vi "BoolDebExample.vi"() -> ()   [LabVIEW 2012]
panel:
  in  "stop":bool
  in  "Default":bool
  out "Boolean 2":bool
  in  "Boolean":bool
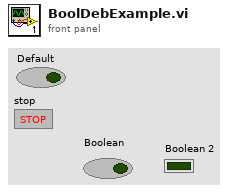
[diagram p1: front panel]
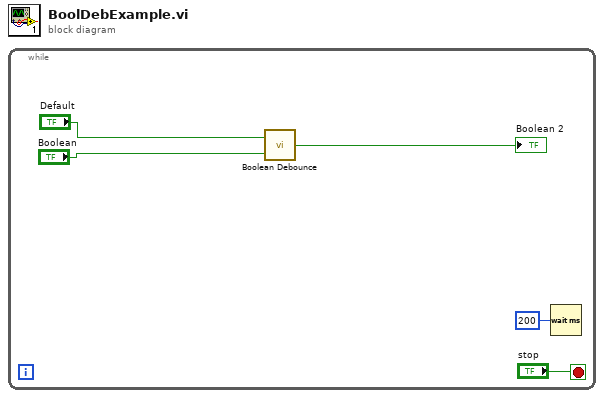
[diagram p0: block diagram]
diagram:
  n1 = while {
    stop <- "stop" stop-if-true
    n2 = call "Boolean Debounce.vi"("Boolean in"="Boolean", "Default"="Default") -> ("Boolean out"=→"Boolean 2":bool)  [unwired: 1 in]
    n3 = Wait (ms)(milliseconds to wait=u32 200) -> ()  [unwired: 1 out]
  }
